vi "PXI-Compute Skip Samples (24-bit only).vi"(5 "AO Sample Rate":dbl, 9 "AI Sample Rate":dbl) -> (4 "Skip Samples":i32)   [LabVIEW 2015]
doc: "Determines the number of AI samples to skip in order to register AO and AI (accounting for the latencies of the 24-bit boards)."
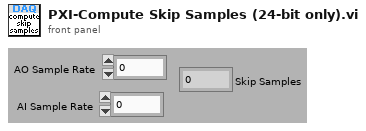
[diagram p1: front panel]
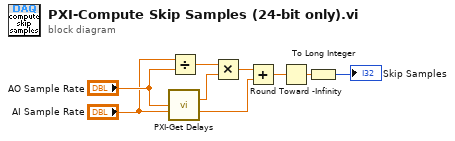
[diagram p0: block diagram]
diagram:
  n1 = call "PXI-Get Delays.vi"("AO Rate (Samples/s)"="AO Sample Rate", "AI Rate (Samples/s)"="AI Sample Rate") -> ("AO delay (samples)"=w4:dbl, "AI delay (samples)"=w3:dbl)  [unwired: 12 in]
  n2 = Divide(x="AI Sample Rate", y="AO Sample Rate") -> (x/y=w5:dbl)
  n3 = Multiply(x=w5, y=w4) -> (x*y=w6:dbl)
  n4 = Add(x=w6, y=w3) -> (x+y=w7:dbl)
  n5 = Round Toward -Infinity(1:w7) -> (0:w8:dbl)
  n6 = To Long Integer(number=w8) -> (32bit integer=→"Skip Samples":i32)
